vi "Get Attribute as JSON.vi"(8 "error in":errorcluster, 10 "Attribute":string="Instruments", 11 "Source":string) -> (0 "error out":errorcluster, 3 "<JSON>":string)   [LabVIEW 2020, in "Instrument Manager.lvclass"]
uses:
  Instrument Manager.lvclass
  Instrument Manager.lvclass/Instrument Manager.ctl
  Config from JSON/Config from JSON.lvclass
  Config from XML/Config from XML.lvclass
  <vilib>/JDP Science/JSONtext/JSONtext.lvlib
  Config from Excel Table/Config from Excel Table.lvclass
  Interfaces/IConfiguration/IConfiguration.lvclass
  Interfaces/IClose/IClose.lvclass
  D:/git/HAL/Source/Config from EXCEL/Config from Excel Table.lvclass
  D:/git/HAL/Source/Interfaces/IClose/IClose.lvclass
  D:/git/HAL/Source/Interfaces/IConfiguration/IConfiguration.lvclass
  D:/git/HAL/Source/Config from XML/Config from XML.lvclass
  D:/git/HAL/Source/Config from JSON/Config from JSON.lvclass
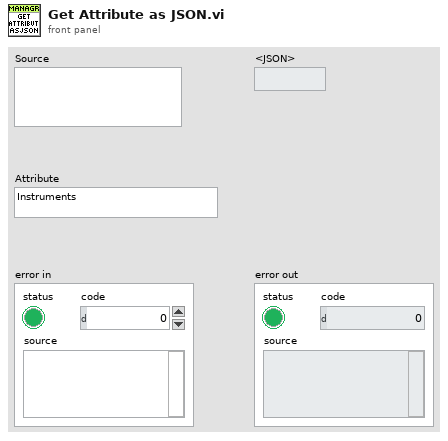
[diagram p1: front panel]
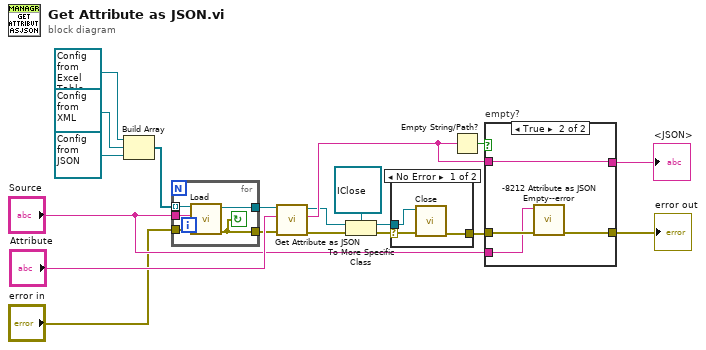
[diagram p0: block diagram]
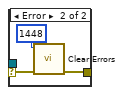
[diagram p2: hidden frame]
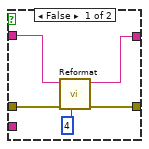
[diagram p3: hidden frame]
diagram:
  n1 = Build Array(refnum<class "Config from Excel Table.lvclass"> refnum ("Config from EXCEL.lvclass"), refnum<class "Config from XML.lvclass"> refnum ("Config from XML.lvclass"), refnum<class "Config from JSON.lvclass"> refnum ("Config from JSON.lvclass")) -> (w17:refnum<class "IConfiguration.lvclass">[])
  n2 = for {
    tunnel: w17 -> [w22] mode=indexing
    tunnel: "Source" -> [w24]
    tunnel: [w23] -> w18
    tunnel: [w21] -> w7
    tunnel: "error in" -> [w20]
    stop <- w21 continue-if-true
    n3 = call-dynamic "Load.vi"("error in"=w20, "Source"=w24, "IConfiguration in"=w22) -> ("error out"=w21:errorcluster, "IConfiguration out"=w23:refnum<class "IConfiguration.lvclass">)  [unwired: 7 in]
  }
  n4 = call-dynamic "Get Attribute as JSON.vi"("error in"=w7, "Attribute"="Attribute", "IConfiguration in"=w18) -> ("error out"=w6:errorcluster, "<JSON>"=w13:string, "IConfiguration out"=w3:refnum<class "IConfiguration.lvclass">)  [unwired: 6 in]
  n5 = To More Specific Class(target class=refnum<class "IClose.lvclass"> refnum ("IClose.lvclass"), reference=w3, error in=w6) -> (specific class reference=w1:refnum<class "IClose.lvclass">, error out=w4:errorcluster)
  n6 = case shown="No Error" w4 {
    selector: w4 -> [w26 w30]
    tunnel: [w27 w29] -> w5
    tunnel: w1 -> [w25 _]
    frame No Error {
      n7 = call-dynamic "Close.vi"("error in"=w26, "IClose in"=w25) -> ("error out"=w27:errorcluster)  [unwired: 8 in, 1 out]
    }
    frame Error {
      n8 = call <vilib>:"Clear Errors.vi"("error in (no error)"=w30, "specific error code to clear (0: all)"=1448) -> ("error out"=w29:errorcluster)  [unwired: 4 in, 1 out]
    }
  }
  n9 = Empty String/Path?(string/path=w13) -> (empty?=w14:bool)
  n10 = case "empty?" shown="True" w14 {
    tunnel: w13 -> [w33 w39]
    tunnel: w5 -> [w35 w38]
    tunnel: [w34 w37] -> w12
    tunnel: [w32 w39] -> w11
    tunnel: "Source" -> [_ w36]
    frame False {
      n11 = call <vilib>:"Reformat.vi"("Pretty Print Levels"=4, "error in (no error)"=w35, "JSON"=w33) -> ("error out"=w34:errorcluster, "<JSON>"=w32:string)  [unwired: 5 in, 2 out]
    }
    frame True {
      n12 = call "-8212 Attribute as JSON Empty--error.vi"("error in"=w38, "Source"=w36) -> ("error out"=w37:errorcluster)  [unwired: 9 in]
    }
  }
  "<JSON>" <- w11
  "error out" <- w12
